vi "Lookup Q.vi"(8 "error in (no error)":errorcluster, 9 "Timeout ms (0)":i32, 10 "Identity":refnum<class "Identity.lvclass">, 11 "VolatusAPI in":refnum<class "VolatusAPI.lvclass">) -> (0 "error out":errorcluster, 2 "MessageQ":refnum<class "MessageQ.lvclass">, 3 "VolatusAPI out":refnum<class "VolatusAPI.lvclass">)   [LabVIEW 2020, in "Volatus.lvlib" / "VolatusAPI.lvclass"]
uses:
  VolatusAPI.lvclass
  Identity/Identity.lvclass
  MessageQ/MessageQ.lvclass
  Q Info.ctl
  VolatusAPI.lvclass/VolatusAPI.ctl
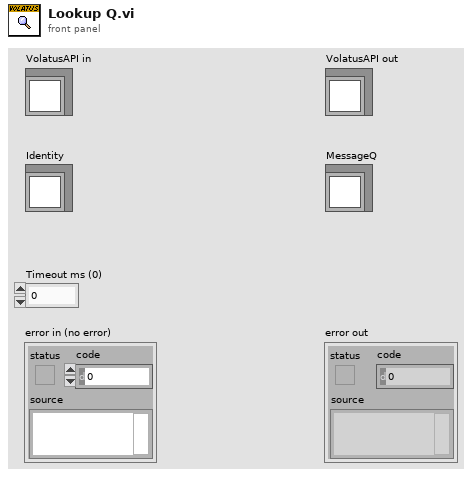
[diagram p1: front panel]
types:
  T1 = typedef "Volatus.lvlib/VolatusAPI.lvclass/Q Info.ctl" = cluster{"Number":i32, "Notifiers":refnum<notifier>[]}
  T2 = typedef "Volatus.lvlib/VolatusAPI.lvclass/MsgQs Ref.ctl" = cluster{"Keys":map{string, T1}, "MsgQs":map{i32, T3}, "Next Number":i32}
  T3 = typedef "Volatus.lvlib/VolatusAPI.lvclass/Registered Q.ctl" = cluster{"Q":refnum<class "MessageQ.lvclass">, "Keys":string[]}
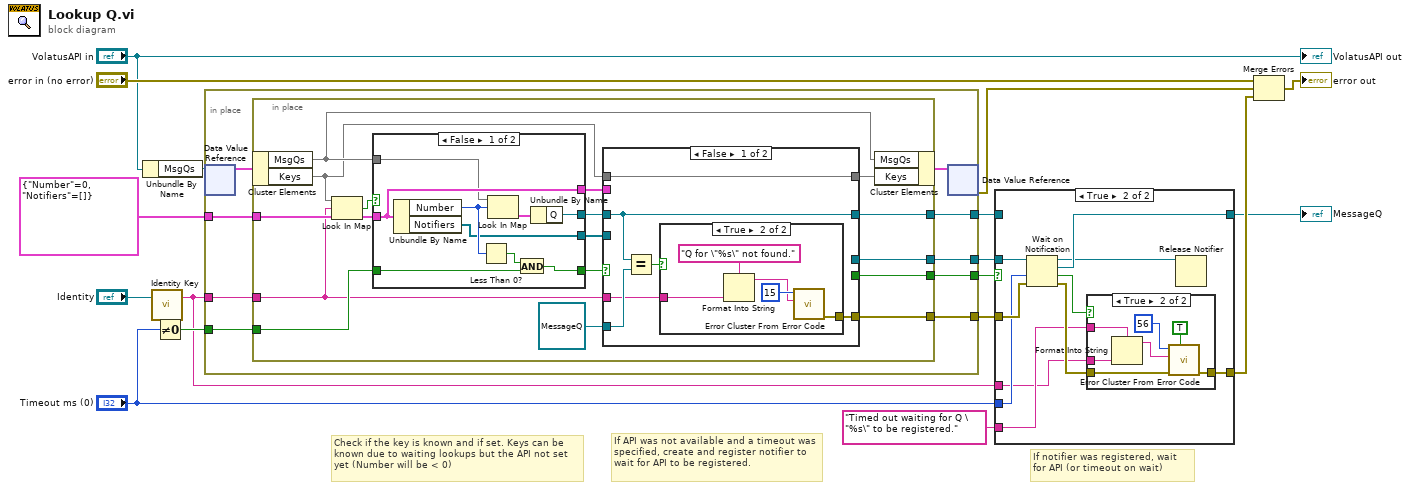
[diagram p0: block diagram]
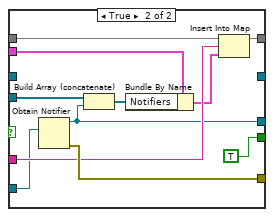
[diagram p4: hidden frame]
diagram:
  # "If notifier was registered, wait for API (or timeout on wait)"
  # "If API was not available and a timeout was specified, create and register notifier to wait for API to be registered."
  # "Check if the key is known and if set. Keys can be known due to waiting lookups but the API not set yet (Number will be < 0)"
  n1 = Unbundle By Name("VolatusAPI in") -> ("MsgQs"=w13:refnum<data-value>)
  n2 = call "Identity Key.vi"("Identity in"="Identity") -> ("Identity Key"=w2:string)  [unwired: 2 in]
  n3 = Not Equal To 0?(x="Timeout ms (0)") -> (x != 0?=w11:bool)
  n4 = in-place {
    in-place-border: w2 -> [w25]
    in-place-border: w11 -> [w24]
    in-place-border: [w23] -> w7
    in-place-border: [w22] -> w8
    in-place-border: [w21] -> w9
    in-place-border: T1 {"Number"=0, "Notifiers"=[]} ("default value") -> [w20]
    in-place-border: [w19] -> w4
    n5 = in-place-dvr #1(w13) -> (w26:T2)  [unwired: 1 out]
    n6 = in-place {
      in-place-border: w25 -> [w34]
      in-place-border: w24 -> [w42]
      in-place-border: [w33] -> w23
      in-place-border: [w30] -> w22
      in-place-border: [w29] -> w21
      in-place-border: w20 -> [w39]
      in-place-border: [w27] -> w19
      n7 = in-place-cluster #2(w26) -> ("MsgQs"=w41:map{i32, T3}, "Keys"=w36:map{string, T1})
      n8 = Look In Map(map=w36, key=w34, default value=w39) -> (key not found?=w43:bool, value=w40:T1)
      n9 = case shown="False" w43 {
        tunnel: w42 -> [w50 w54]
        tunnel: w41 -> [w44 _]
        tunnel: w40 -> [w45 w53]
        tunnel: [w52 _] -> w37
        tunnel: [w47 w54] -> w38
        tunnel: [w46 _] -> w32
        tunnel: [w45 w53] -> w31
        frame False {
          n10 = Unbundle By Name(w45) -> ("Number"=w51:i32, "Notifiers"=w46:refnum<notifier>[])
          n11 = Less Than 0?(x=w51) -> (x < 0?=w49:bool)
          n12 = Look In Map(map=w44, key=w51) -> (value=w48:T3)  [unwired: 1 in, 1 out]
          n13 = And(x=w49, y=w50) -> (x .and. y?=w47:bool)
          n14 = Unbundle By Name(w48) -> ("Q"=w52:refnum<class "MessageQ.lvclass">)
        }
        frame True {
        }
      }
      n15 = case shown="False" w38 {
        tunnel: w37 -> [w59 _]
        tunnel: w36 -> [w60 w72]
        tunnel: [w60 w71] -> w35
        tunnel: w34 -> [w55 w70]
        tunnel: [w59 _] -> w33
        tunnel: w32 -> [_ w75]
        tunnel: w31 -> [_ w74]
        tunnel: [_ w68] -> w30
        tunnel: [_ TRUE] -> w29
        tunnel: refnum<class "MessageQ.lvclass"> refnum ("Volatus:MessageQ") -> [w58 w66]
        tunnel: [w56 w76] -> w27
        frame False {
          n16 = Equal?(x=w59, y=w58) -> (x = y?=w57:bool)
          n17 = case shown="True" w57 {
            tunnel: [_ w65] -> w56
            tunnel: w55 -> [_ w62]
            frame False {
            }
            frame True {
              n18 = Format Into String(format string="Q for \"%s\" not found.", w62) -> (resulting string=w61:string)  [unwired: 2 in, 1 out]
              n19 = call <vilib>:"Error Cluster From Error Code.vi"("error message (\"\")"=w61, "error code (0)"=15) -> ("error out"=w65:errorcluster)  [unwired: 7 in]
            }
          }
        }
        frame True {
          n20 = Obtain Notifier(notification data type=w66) -> (notifier out=w68:refnum<notifier>, error out=w76:errorcluster)  [unwired: 3 in, 1 out]
          n21 = Build Array (concatenate)(w75, w68) -> (w73:refnum<notifier>[])
          n22 = Bundle By Name(cluster=w74, "Notifiers"=w73) -> (w69:T1)
          n23 = Insert Into Map(map in=w72, key=w70, value=w69) -> (map out=w71:map{string, T1})  [unwired: 2 out]
        }
      }
      n24 = in-place-cluster #2("MsgQs"=w41, "Keys"=w35) -> (w18:T2)
    }
    n25 = in-place-dvr #1(w18) -> (w16:errorcluster)  [unwired: 1 out]
  }
  n26 = case shown="True" w9 {
    tunnel: w8 -> [_ w87]
    tunnel: w7 -> [w78 _]
    tunnel: [w78 w86] -> w1
    tunnel: "Timeout ms (0)" -> [_ w85]
    tunnel: w4 -> [w77 w88]
    tunnel: [w77 w81] -> w17
    tunnel: "Timed out waiting for Q \"%s\" to be registered." -> [_ w80]
    tunnel: w2 -> [_ w79]
    frame False {
    }
    frame True {
      n27 = Wait on Notification(notifier=w87, timeout in ms (-1)=w85, error in (no error)=w88) -> (notifier out=w84:refnum<notifier>, notification=w86:refnum<class "MessageQ.lvclass">, timed out?=w83:bool, error out=w82:errorcluster)  [unwired: 1 in]
      n28 = case shown="True" w83 {
        tunnel: w82 -> [w89 w96]
        tunnel: [w89 w94] -> w81
        tunnel: w80 -> [_ w91]
        tunnel: w79 -> [_ w90]
        frame False {
        }
        frame True {
          n29 = Format Into String(format string=w91, w90) -> (resulting string=w93:string)  [unwired: 2 in, 1 out]
          n30 = call <vilib>:"Error Cluster From Error Code.vi"("show call chain? (False)"=TRUE, "error in (no error)"=w96, "error message (\"\")"=w93, "error code (0)"=56) -> ("error out"=w94:errorcluster)  [unwired: 5 in]
        }
      }
      n31 = Release Notifier(notifier=w84) -> ()  [unwired: 2 in, 3 out]
    }
  }
  "MessageQ" <- w1
  n32 = Merge Errors("error in (no error)", w16, w17) -> (→"error out":errorcluster)
  "VolatusAPI out" <- "VolatusAPI in"
